vi "Initialize.vi"(8 "error in":errorcluster, 11 "Shared Resources in":refnum<class "Shared Resources.lvclass">) -> (0 "error out":errorcluster, 3 "Shared Resources out":refnum<class "Shared Resources.lvclass">)   [LabVIEW 2020, in "AIM ARINC 664 Engine.lvlib" / "Implementation.lvlib" / "Shared Resources.lvclass"]
uses:
  Shared Resources.lvclass
  Program Files/National Instruments/LabVIEW 2024/instr.lib/AIM GmbH/_AIM 664/AIM664LV.lvlib
  Program Files/National Instruments/LabVIEW 2024/instr.lib/AIM GmbH/_AIM 664/bsp/Fdx Create Session (Generic-Board).vi
  <vilib>/Utility/sysdir.llb/System Directory Type.ctl
  <vilib>/Utility/SystemLogging/NI_SystemLogging.lvlib
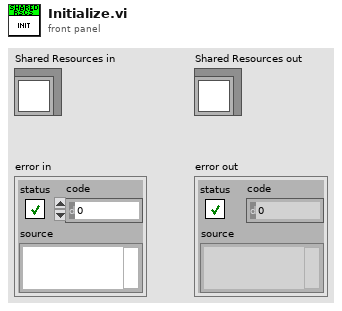
[diagram p1: front panel]
types:
  T1 = typedef "AIM664LV.lvlib/port_speed.ctl" = u32
  T2 = cluster{"[0]":u32, "[1]":u32, "[2]":u32, "[3]":u32}
  T3 = typedef "System Directory Type.ctl" = i32
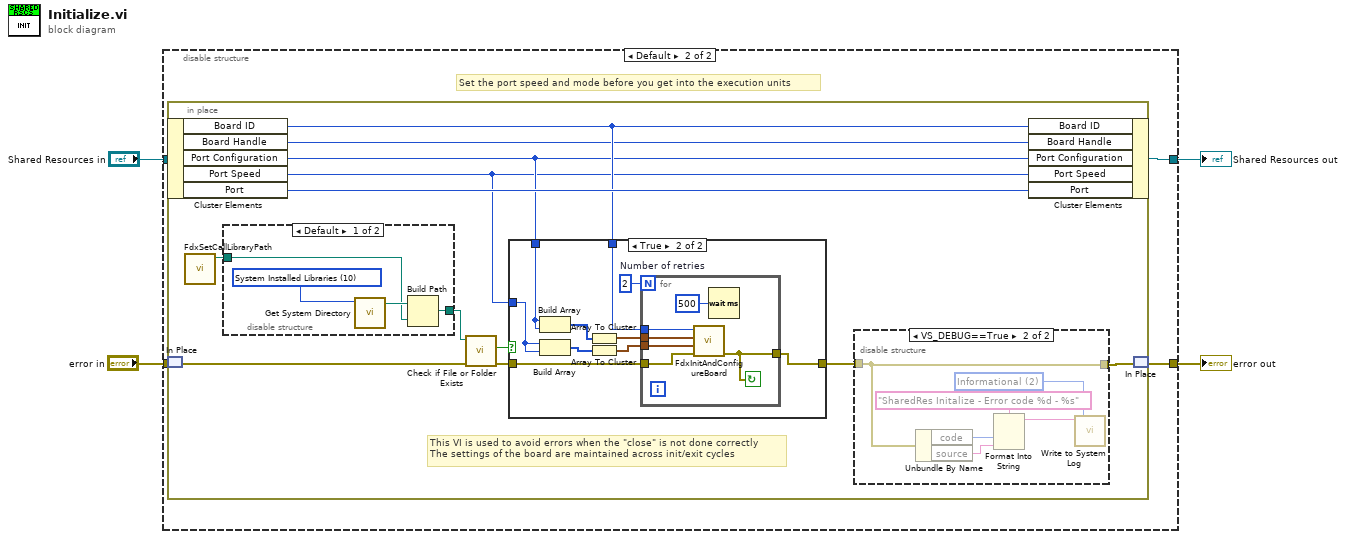
[diagram p0: block diagram]
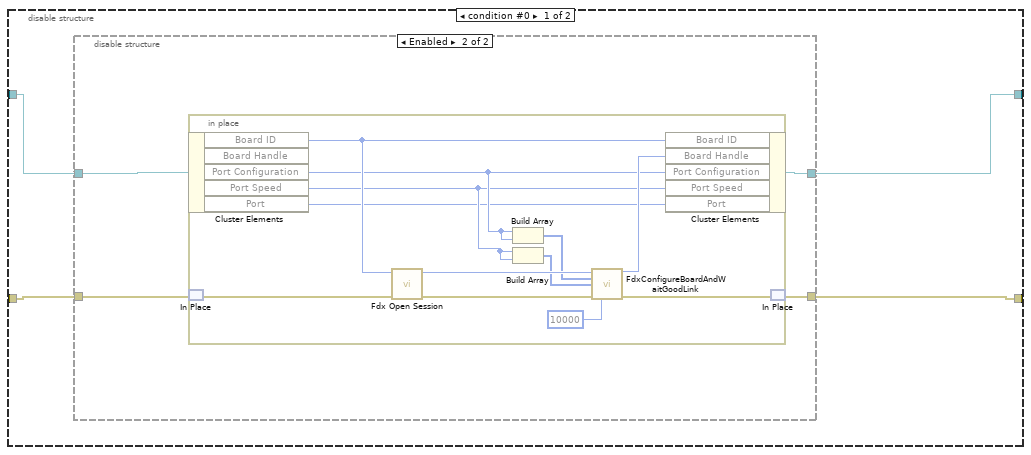
[diagram p2: hidden frame]
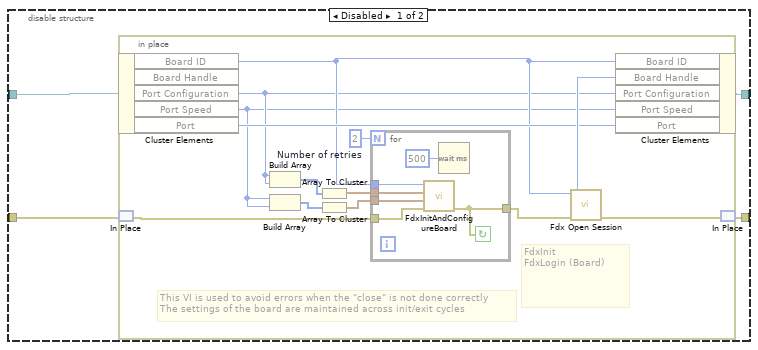
[diagram p3: hidden frame]
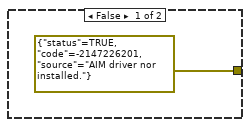
[diagram p6: hidden frame]
diagram:
  n1 = disable-structure shown="Default" {
    disable-tunnel: "Shared Resources in" -> [w8 w51]
    disable-tunnel: [w7 w50] -> w3
    disable-tunnel: "error in" -> [w6 w48]
    disable-tunnel: [w5 w49] -> w1
    frame condition #0 {
      n2 = disable-structure shown="Enabled" {
        disable-tunnel: w8 -> [w12 w33]
        disable-tunnel: [w11 w32] -> w7
        disable-tunnel: w6 -> [w10 w35]
        disable-tunnel: [w9 w34] -> w5
        frame Disabled {
          n3 = in-place {
            w22 = 2  # Number of retries
            # "FdxInit\nFdxLogin (Board)"
            # "This VI is used to avoid errors when the \"close\" is not done correctly\nThe settings of the board are maintained across init/exit cycles"
            n4 = in-place-cluster #1(w12) -> ("Board ID"=w20:i32, "Port Configuration"=w19:u32, "Port Speed"=w17:T1, "Port"=w23:i32)  [unwired: 1 out]
            n5 = in-place-match #2(w10) -> (w14:errorcluster)
            n6 = Build Array(w19, w19) -> (w18:u32[])
            n7 = Build Array(w17, w17) -> (w16:T1[])
            n8 = Array To Cluster(array=w18) -> (cluster=w21:T2)
            n9 = Array To Cluster(array=w16) -> (cluster=w15:cluster{"[0]":T1, "[1]":T1, "[2]":T1, "[3]":T1})
            n10 = for {
              N: w22 -> [_]
              tunnel: [w30] -> w13
              tunnel: w20 -> [w29]
              tunnel: w21 -> [w28]
              tunnel: w15 -> [w27]
              tunnel: w14 -> [w26]
              stop <- w30 continue-if-true
              n11 = call "FdxInitAndConfigureBoard.vi"("error in (no error)"=w26, "PortSpeed (100Mbit)"=w27, "PortConfig (single)"=w28, "board index"=w29) -> ("error out"=w30:errorcluster)  [unwired: 3 in, 4 out]
              n12 = Wait (ms)(milliseconds to wait=u32 500) -> ()  [unwired: 1 out]
            }
            n13 = call-poly "Fdx Open Session.vi"("error in (no error)"=w13, "board"=w20) -> ("error out"=w25:errorcluster, "InstrumentHandle_board out"=w24:u32)  [unwired: 7 in, 1 out]
            n14 = in-place-cluster #1("Board ID"=w20, "Board Handle"=w24, "Port Configuration"=w19, "Port Speed"=w17, "Port"=w23) -> (w11:refnum<class "Shared Resources.lvclass">)
            n15 = in-place-match #2(w25) -> (w9:errorcluster)
          }
        }
        frame Enabled {
          n16 = in-place {
            n17 = in-place-cluster #3(w33) -> ("Board ID"=w47:i32, "Port Configuration"=w38:u32, "Port Speed"=w37:T1, "Port"=w36:i32)  [unwired: 1 out]
            n18 = in-place-match #4(w35) -> (w42:errorcluster)
            n19 = call-poly "Fdx Open Session.vi"("error in (no error)"=w42, "board"=w47) -> ("error out"=w46:errorcluster, "InstrumentHandle_board out"=w45:u32)  [unwired: 7 in, 1 out]
            n20 = Build Array(w38, w38) -> (w40:u32[])
            n21 = Build Array(w37, w37) -> (w39:T1[])
            n22 = call "FdxConfigureBoardAndWaitGoodLink.vi"("InstrumentHandle_board in"=w45, "PortConfig"=w40, "PortSpeed"=w39, "error in"=w46, "timeout (ms)"=u32 10000) -> ("InstrumentHandle_board out"=w44:u32, "error out"=w43:errorcluster)  [unwired: 7 in, 2 out]
            n23 = in-place-cluster #3("Board ID"=w47, "Board Handle"=w44, "Port Configuration"=w38, "Port Speed"=w37, "Port"=w36) -> (w32:refnum<class "Shared Resources.lvclass">)
            n24 = in-place-match #4(w43) -> (w34:errorcluster)
          }
        }
      }
    }
    frame condition #1 (active) {
      # "Set the port speed and mode before you get into the execution units"
      n25 = in-place {
        # "This VI is used to avoid errors when the \"close\" is not done correctly\nThe settings of the board are maintained across init/exit cycles"
        n26 = in-place-cluster #5(w51) -> ("Board ID"=w62:i32, "Board Handle"=w59:i32, "Port Configuration"=w61:u32, "Port Speed"=w60:T1, "Port"=w63:i32)
        n27 = in-place-match #6(w48) -> (w58:errorcluster)
        n28 = call "FdxSetCallLibraryPath.vi"() -> ("DllPath"=w55:path)  [unwired: 11 in]
        n29 = disable-structure shown="Default" {
          disable-tunnel: w55 -> [w72 w75]
          disable-tunnel: [w71 w75] -> w54
          frame condition #0 (active) {
            w74 = T3 10 items=["User Home"=0, "User Desktop"=1, "User Documents"=2, "User Application Data"=3, "User Preferences"=4, "User Temporary"=5, "Public Documents"=6, "Public Application Data"=7, "Public Preferences"=8, "Public Cache"=13, "System Core Libraries"=9, "System Installed Libraries"=10, "Application Files"=11, "Boot Volume Root"=12] ("system directory type")
            n30 = call <vilib>:"Get System Directory.vi"("system directory type"=w74) -> ("system directory"=w73:path)  [unwired: 10 in]
            n31 = Build Path(base path=w73, name or relative path=w72) -> (appended path=w71:path)
          }
          frame condition #1 {
          }
        }
        n32 = call <vilib>:"Check if File or Folder Exists.vi"("error in (no error)"=w58, "path"=w54) -> ("error out"=w57:errorcluster, "file or folder exists?"=w56:bool)  [unwired: 7 in, 1 out]
        n33 = case shown="True" w56 {
          tunnel: w62 -> [_ w84]
          tunnel: w61 -> [_ w83]
          tunnel: w60 -> [_ w81]
          tunnel: [errorcluster {"status"=TRUE, "code"=-2147226201, "source"="AIM driver nor installed."} ("error out") w78] -> w53
          tunnel: w57 -> [_ w77]
          frame False {
          }
          frame True {
            w86 = 2  # Number of retries
            n34 = Build Array(w83, w83) -> (w82:u32[])
            n35 = Build Array(w81, w81) -> (w80:T1[])
            n36 = Array To Cluster(array=w82) -> (cluster=w85:T2)
            n37 = Array To Cluster(array=w80) -> (cluster=w79:cluster{"[0]":T1, "[1]":T1, "[2]":T1, "[3]":T1})
            n38 = for {
              N: w86 -> [_]
              tunnel: [w91] -> w78
              tunnel: w84 -> [w90]
              tunnel: w85 -> [w89]
              tunnel: w79 -> [w88]
              tunnel: w77 -> [w87]
              stop <- w91 continue-if-true
              n39 = call "FdxInitAndConfigureBoard.vi"("error in (no error)"=w87, "PortSpeed (100Mbit)"=w88, "PortConfig (single)"=w89, "board index"=w90) -> ("error out"=w91:errorcluster)  [unwired: 3 in, 4 out]
              n40 = Wait (ms)(milliseconds to wait=u32 500) -> ()  [unwired: 1 out]
            }
          }
        }
        n41 = disable-structure shown="VS_DEBUG==True" {
          disable-tunnel: w53 -> [w64 w65]
          disable-tunnel: [w64 w65] -> w52
          frame condition #0 (active) {
          }
          frame condition #1 {
            w68 = 2 items=["Error", "Warning", "Informational"] ("severity")
            n42 = Unbundle By Name(w65) -> ("code"=w67:i32, "source"=w66:string)
            n43 = Format Into String(format string="SharedRes Initalize - Error code %d - %s", w67, w66) -> (resulting string=w69:string)  [unwired: 2 in, 1 out]
            n44 = call <vilib>:"Write to System Log.vi"("severity"=w68, "message"=w69) -> ()  [unwired: 9 in, 1 out]
          }
        }
        n45 = in-place-cluster #5("Board ID"=w62, "Board Handle"=w59, "Port Configuration"=w61, "Port Speed"=w60, "Port"=w63) -> (w50:refnum<class "Shared Resources.lvclass">)
        n46 = in-place-match #6(w52) -> (w49:errorcluster)
      }
    }
  }
  "error out" <- w1
  "Shared Resources out" <- w3
